vi "closeMotor.vi"(2 ".NET Refnum in":refnum<k24>) -> ()   [LabVIEW 2021]
doc: "André Romero - 2017\nandretec@ifsc.usp.br"
uses:
  C:/user-Lab/AndreTec/GITs/andretec/Thorlabs-Vector-Move/kinesisTec/Kinesis/Thorlabs.MotionControl.Controls.dll
  Kinesis/Thorlabs.MotionControl.Controls.dll
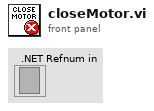
[diagram p1: front panel]
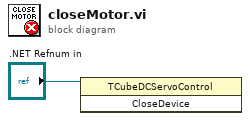
[diagram p0: block diagram]
diagram:
  n1 = invoke class="TCubeDCServoControl" method="CloseDevice"(reference=".NET Refnum in") -> ()  [unwired: 2 in, 3 out]
